vi "Analog Input Timing.vi"() -> ()   [LabVIEW 2010]
uses:
  <vilib>/eio/EIONode/EIONode.xnode
  <vilib>/rvi/eio/nirviEIOImplementation/nirviEIOImplementation.xnode
  <vilib>/rvi/eio/common/nirviEmuClasses.ctl
  <vilib>/rvi/eio/common/nirviEmuTemplateMethod_noerrors.vi
panel:
  in  "Limit":i16
  out "Over Limit":bool
  out "Connector0/AI0":i16
  in  "AI Sample Time (ms)":u32=500
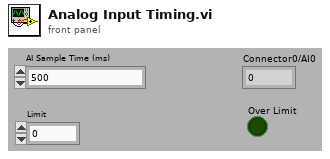
[diagram p1: front panel]
types:
  T1 = typedef "nirviEmuClasses.ctl" = enum16{"IO Read", "IO Write", "Method", "Property Read", "Property Write"}
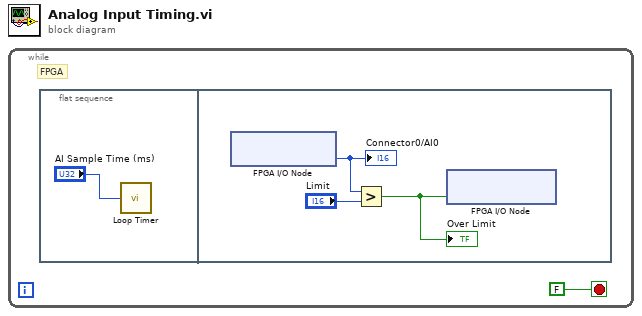
[diagram p0: block diagram]
diagram:
  n1 = while {
    stop <- FALSE stop-if-true
    # "FPGA"
    n2 = flat-sequence {
      frame #0 {
        n3 = call "Loop Timer"("Count(mSec)"="AI Sample Time (ms)") -> ()  [unwired: 1 out]
      }
      frame #1 {
        n4 = xnode "FPGA I/O Node"() -> ("Analog Input"=w5:i16)  [unwired: 1 in, 1 out]
        "Connector0/AI0" <- w5
        n5 = Greater?(x=w5, y="Limit") -> (0:w3:bool)
        "Over Limit" <- w3
        n6 = xnode "FPGA I/O Node"("Digital Output"=w3) -> ()  [unwired: 1 in, 1 out]
      }
    }
  }
